vi "WriteJson.vi"(8 "error in (no error)":errorcluster, 10 "JSON string":string, 11 "Web Request in":refnum<class "Web Request.lvclass">) -> (0 "error out":errorcluster, 3 "Web Request out":refnum<class "Web Request.lvclass">)   [LabVIEW 2014, in "FRCts20_WebMethods.lvlib"]
uses:
  FRCts20_WebMethods.lvlib
  <vilib>/wsapi/Web Request.lvclass
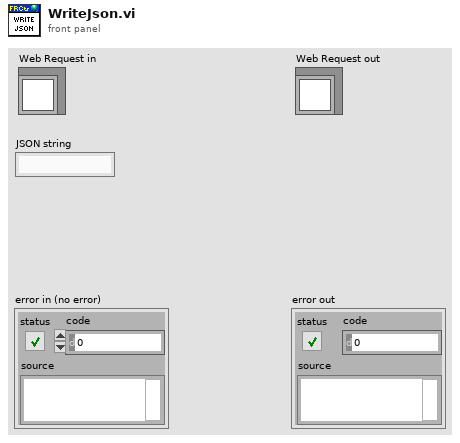
[diagram p1: front panel]
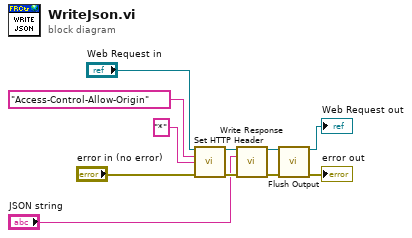
[diagram p0: block diagram]
diagram:
  n1 = call <vilib>:"Set HTTP Header.vi"("LabVIEW Web Service Request"="Web Request in", "header"="Access-Control-Allow-Origin", "header value"="*", "error in (no error)"="error in (no error)") -> ("LabVIEW Web Service Request out"=w11:refnum<class "Web Request.lvclass">, "error out"=w9:errorcluster)  [unwired: 10 in]
  n2 = call <vilib>:"Write Response.vi"("LabVIEW Web Service Request"=w11, "response string"="JSON string", "error in (no error)"=w9) -> ("LabVIEW Web Service Request out"=w4:refnum<class "Web Request.lvclass">, "error out"=w3:errorcluster)  [unwired: 11 in]
  n3 = call <vilib>:"Flush Output.vi"("LabVIEW Web Service Request"=w4, "error in (no error)"=w3) -> ("LabVIEW Web Service Request out"=→"Web Request out":refnum<class "Web Request.lvclass">, "error out"=→"error out":errorcluster)  [unwired: 12 in]
